vi "Sensor name to SensorID.vi"(7 "Sensor name":string) -> (0 "Sensor Name Only":string, 1 "Database Connection":T1, 3 "Column Names":string[](array[string]), 4 "TableNameArray":string[](array[string]), 5 "Time Name":string, 6 "Modulus Number":string)   [LabVIEW 2010, in "SQL project lib.lvlib"]
uses:
  LabView Dec.8/LabView Dec.8/SQL project lib.lvlib
  <vilib>/addons/database/Connection.llb/Conn ObjectReference.ctl
  SubVi's/DAQ Connection Variable.vi
  LabView Dec.8/LabView Dec.8/SubVi's/Connection Variable 1.vi
  <vilib>/addons/database/NI_Database_API.lvlib
panel:
  # "Takes Sensor name and Local ID, separates them and outputs Name\nand Absolute ID"
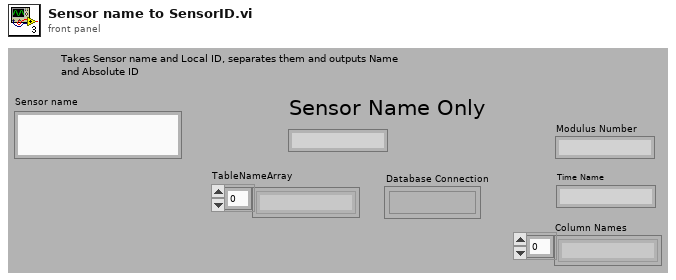
[diagram p1: front panel]
types:
  T1 = typedef "NI_Database_API.lvlib/Conn ObjectReference.ctl" = refnum<k1>
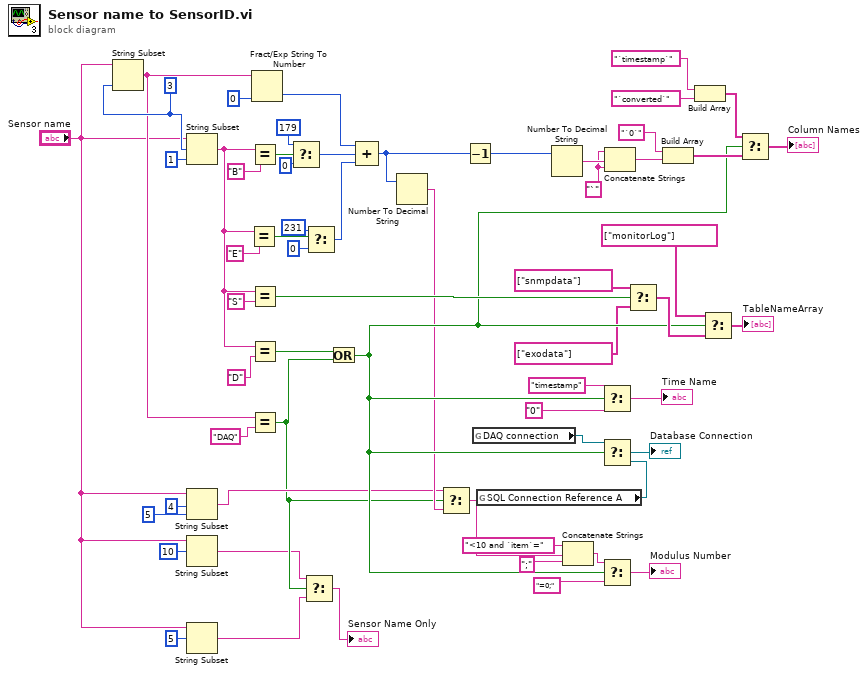
[diagram p0: block diagram]
diagram:
  w30 = "`" ("string")
  w60 = 3 ("length (rest)")
  n1 = String Subset(string="Sensor name", length (rest)=w60) -> (substring=w15:string)  [unwired: 1 out]
  n2 = String Subset(string="Sensor name", offset (0)=w60, length (rest)=1 ("length (rest)")) -> (substring=w42:string)
  n3 = String Subset(string="Sensor name", offset (0)=4 ("length (rest)"), length (rest)=5 ("length (rest)")) -> (substring=w9:string)
  n4 = String Subset(string="Sensor name", offset (0)=10) -> (substring=w3:string)  [unwired: 1 out]
  n5 = String Subset(string="Sensor name", offset (0)=5) -> (substring=w7:string)  [unwired: 1 out]
  n6 = Equal?(x=w42, y="E") -> (x = y?=w50:bool)
  n7 = Equal?(x=w42, y="B") -> (x = y?=w49:bool)
  n8 = Equal?(x=w42, y="S") -> (x = y?=w46:bool)
  n9 = Equal?(x=w42, y="D") -> (x = y?=w16:bool)
  n10 = Equal?(x=w15, y="DAQ") -> (x = y?=w8:bool)
  n11 = Fract/Exp String To Number(string=w15, default (0 dbl)=0) -> (number=w52:i32)  [unwired: 3 out]
  n12 = Select(t=179, s=w49, f=0) -> (s? t:f=w56:i32)
  n13 = Select(t=w3, s=w8, f=w7) -> (s? t:f=→"Sensor Name Only":string)
  n14 = Select(t=231, s=w50, f=0) -> (s? t:f=w48:i32)
  n15 = Or(x=w16, y=w8) -> (x .or. y?=w17:bool)
  n16 = Compound Arithmetic op=ADD(w52, w56, w48) -> (w19:i32)
  n17 = Number To Decimal String(number=w19) -> (decimal integer string=w13:string)  [unwired: 1 out]
  n18 = Select(t=w9, s=w8, f=w13) -> (s? t:f=w12:string)
  n19 = Decrement(x=w19) -> (x-1=w20:i32)
  n20 = global read "DAQ Connection Variable.vi" "DAQ connection"() -> (w38:T1)
  n21 = global read "Connection Variable 1.vi" "SQL Connection Reference A"() -> (w2:T1)
  n22 = Number To Decimal String(number=w20) -> (decimal integer string=w31:string)  [unwired: 1 out]
  n23 = Concatenate Strings("<10 and `item`=", w12, ";") -> (w21:string)
  n24 = Select(t="timestamp", s=w17, f="0") -> (s? t:f=→"Time Name":string)
  n25 = Select(t=w38, s=w17, f=w2) -> (s? t:f=→"Database Connection":T1)
  n26 = Select(t=w21, s=w17, f="=0;") -> (s? t:f=→"Modulus Number":string)
  n27 = Concatenate Strings(w30, w31, w30) -> (w29:string)
  n28 = Select(t=string[] ["snmpdata"], s=w46, f=string[] ["exodata"]) -> (s? t:f=w41:string[])
  n29 = Build Array("`0`" ("element"), w29) -> (w27:string[])
  n30 = Build Array("`timestamp`" ("element"), "`converted`" ("element")) -> (w24:string[])
  n31 = Select(t=string[] ["monitorLog"], s=w17, f=w41) -> (s? t:f=→"TableNameArray":string[])
  n32 = Select(t=w24, s=w17, f=w27) -> (s? t:f=→"Column Names":string[])
